vi "init.vi"(8 "error in":errorcluster, 10 "TBM module configuration in":refnum<class "TBM module configuration.lvclass">, 11 "fixed channel runtime in":refnum<class "control module runtime.lvclass">) -> (0 "error out":errorcluster, 1 "data allocations":T1, 2 "execution settings":T4, 3 "fixed channel runtime out":refnum<class "control module runtime.lvclass">)   [LabVIEW 2013, in "control module runtime.lvclass"]
doc: "Provides an interface for initializing a module at runtime. While this interface performs no operations, a child should provide an override which may open any necessary references or sessions, allocate necessary memory, and perform any final configuration validataion before providing the full configuration <b>execution data</b> to the calling process."
uses:
  control module runtime.lvclass
  <vilib>/NI/Tag Bus Module Framework/module configuration/TBM module configuration.lvclass
  <vilib>/NI/Tag Bus Module Framework/runtime/execution settings.ctl
  <vilib>/NI/Tag Bus Module Framework/channel/data tables.ctl
  <vilib>/NI/Tag Bus/dictionary/data dictionary.lvclass
  <vilib>/NI/Tag Bus/dictionary table pair.ctl
  <vilib>/NI/Tag Bus/table/data table.ctl
  configuration/control module configuration.lvclass
  <vilib>/NI/Tag Bus Module Framework/channel/TBM channel.lvclass
  <vilib>/NI/Tag Bus Module Framework/runtime/TBM module execution interface.lvclass
  <vilib>/NI/Tag Bus/tag bus.lvlib
  <vilib>/NI/Tag Bus/table/data table.lvlib
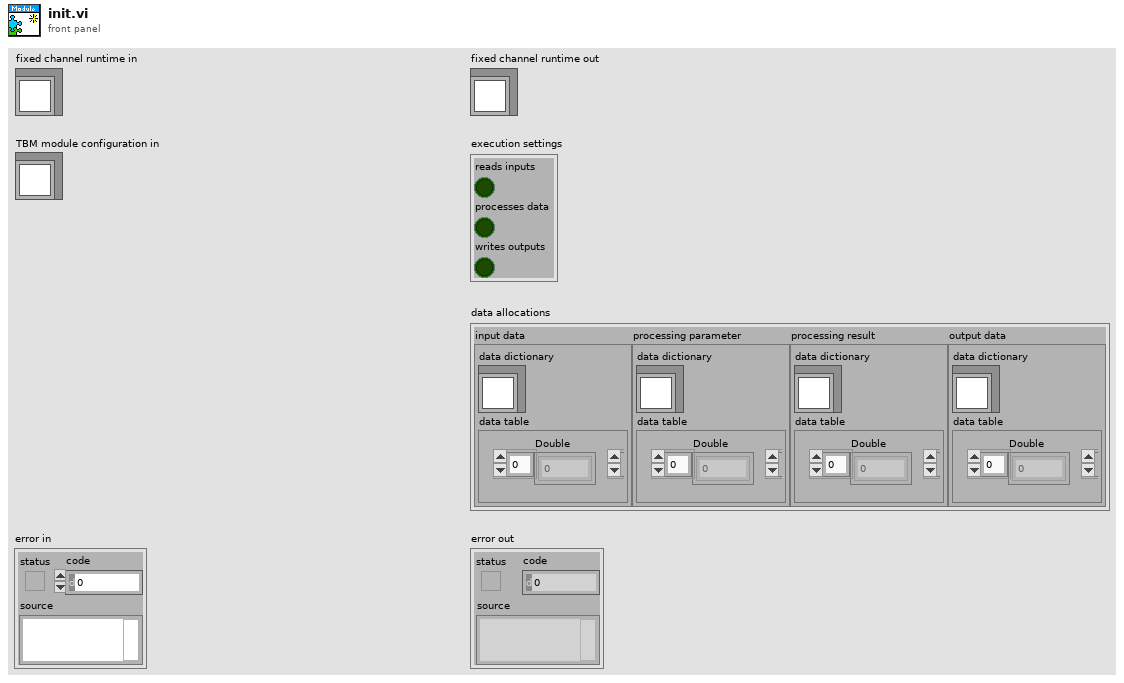
[diagram p1: front panel]
types:
  T1 = typedef "TBM channel.lvclass/data tables.ctl" = cluster{"input data":T2, "processing parameter":T2, "processing result":T2, "output data":T2}
  T2 = typedef "tag bus.lvlib/dictionary table pair.ctl" = cluster{"data dictionary":refnum<class "data dictionary.lvclass">, "data table":T3}
  T3 = typedef "tag bus.lvlib/data table.lvlib/data table.ctl" = cluster{"Double":dbl[], "Single":sgl[], "I64":i64[], "I32":i32[], "I16":i16[], "I8":i8[], "U64":u64[], "U32":u32[], "U16":u16[], "U8":u8[], "Boolean":bool[], "String":string[], "Array of Double":cluster{"DBL Array":dbl[]}[], "Array of Single":cluster{"SGL Array":sgl[]}[], "Array of I64":cluster{"I64 Array":i64[]}[], "Array of I32":cluster{"I32 Array":i32[]}[], "Array of I16":cluster{"I16 Array":i16[]}[], "Array of I8":cluster{"I8 Array":i8[]}[], "Array of U64":cluster{"U64 Array":u64[]}[], "Array of U32":cluster{"U32 Array":u32[]}[], "Array of U16":cluster{"U16 Array":u16[]}[], "Array of U8":cluster{"U8 Array":u8[]}[], "Array of Boolean":cluster{"Boolean Array":bool[]}[], "Array of String":cluster{"String Array":string[]}[]}
  T4 = typedef "TBM module execution interface.lvclass/execution settings.ctl" = cluster{"reads inputs":bool, "processes data":bool, "writes outputs":bool}
  T5 = typedef "control module runtime.lvclass/Channel Run Time Mapping Info.ctl" = cluster{"Channel Indicies":i32[], "Channel Names":string[]}
  T6 = typedef "TBM channel.lvclass/channel classification.ctl" = enum16{"input data", "output data", "processing parameter", "processing result"}
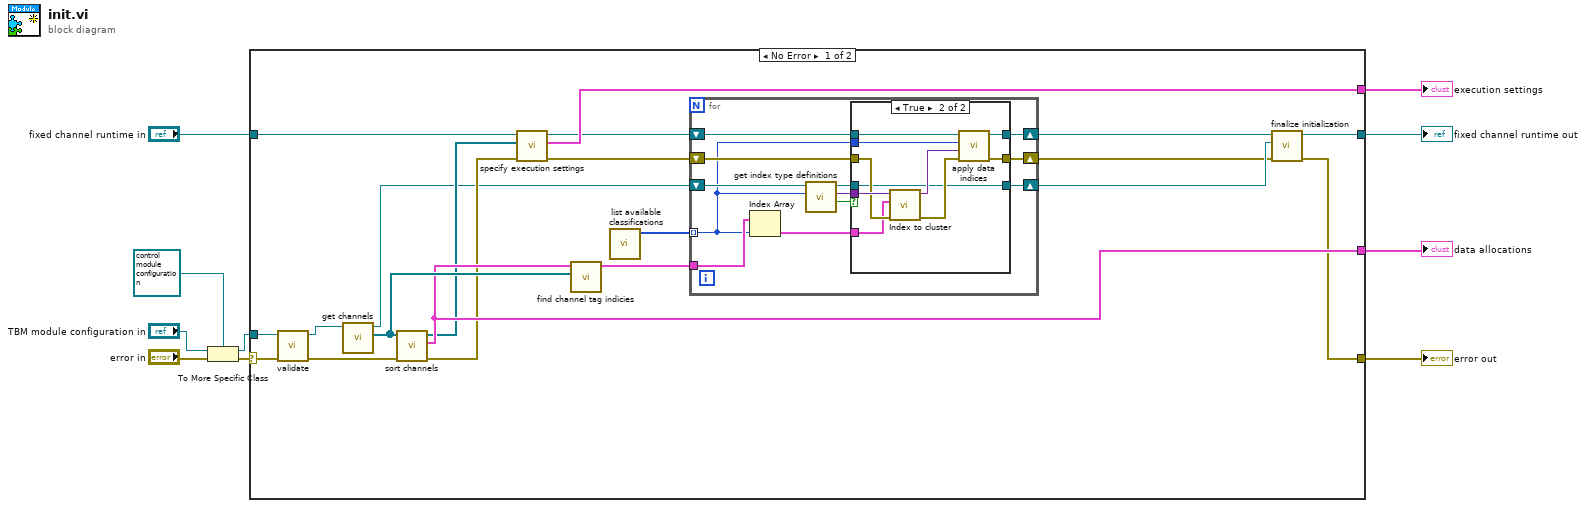
[diagram p0: block diagram]
diagram:
  n1 = To More Specific Class(target class=refnum<class "control module configuration.lvclass"> refnum ("Synchronous module configuration"), reference="TBM module configuration in", error in="error in") -> (specific class reference=w1:refnum<class "control module configuration.lvclass">, error out=w2:errorcluster)
  n2 = case shown="No Error" w2 {
    selector: w2 -> [w29 w56]
    tunnel: w1 -> [w28 _]
    tunnel: "fixed channel runtime in" -> [w22 w57]
    tunnel: [w24 w57] -> w8
    tunnel: [w23 w56] -> w7
    tunnel: [w25 _] -> w5
    tunnel: [w21 _] -> w6
    frame No Error {
      n3 = call-dynamic "validate.vi"("error in"=w29, "fixed channel configuration in"=w28) -> ("error out"=w30:errorcluster, "fixed channel configuration out"=w27:refnum<class "control module configuration.lvclass">)  [unwired: 8 in]
      n4 = call-dynamic "get channels.vi"("fixed channel configuration in"=w27) -> ("channels"=w26:refnum<class "TBM channel.lvclass">[], "fixed channel configuration out"=w16:refnum<class "control module configuration.lvclass">)  [unwired: 9 in]
      n5 = call <vilib>:"sort channels.vi"("error in"=w30, "channels in"=w26) -> ("error out"=w19:errorcluster, "data allocations"=w25:T1, "channels out"=w20:refnum<class "TBM channel.lvclass">[])  [unwired: 7 in]
      n6 = call-dynamic "specify execution settings.vi"("error in"=w19, "channels"=w20, "fixed channel runtime in"=w22) -> ("error out"=w12:errorcluster, "execution settings"=w21:T4, "fixed channel runtime out"=w18:refnum<class "control module runtime.lvclass">)  [unwired: 6 in]
      n7 = call "find channel tag indicies.vi"("channels"=w26, "data allocations"=w25) -> ("classified indices"=w11:T5[])  [unwired: 9 in]
      n8 = call <vilib>:"list available classifications.vi"() -> ("supported types"=w17:T6[])  [unwired: 11 in]
      n9 = for {
        shift-right: [w38] -> w15
        shift-left: w18 -> [w37]
        tunnel: w17 -> [w32] mode=indexing
        shift-right: [w39] -> w14
        shift-left: w16 -> [w42]
        shift-right: [w36] -> w13
        shift-left: w12 -> [w35]
        tunnel: w11 -> [w33]
        n10 = Index Array(array=w33, index=w32) -> (element=w31:T5)
        n11 = call-dynamic "get index type definitions.vi"("channel classification"=w32, "fixed channel configuration in"=w42) -> ("valid?"=w41:bool, "index cluster"=w34:variant, "fixed channel configuration out"=w40:refnum<class "control module configuration.lvclass">)  [unwired: 7 in]
        n12 = case shown="True" w41 {
          tunnel: w40 -> [w45 w47]
          tunnel: [w45 w47] -> w39
          tunnel: [w44 w55] -> w38
          tunnel: w37 -> [w44 w54]
          tunnel: [w43 w53] -> w36
          tunnel: w35 -> [w43 w50]
          tunnel: w32 -> [_ w52]
          tunnel: w34 -> [_ w51]
          tunnel: w31 -> [_ w46]
          frame False {
          }
          frame True {
            n13 = call "Index to cluster.vi"("error in"=w50, "Input Mapping Info"=w46, "Variant in"=w51) -> ("error out"=w49:errorcluster, "Variant out"=w48:variant)  [unwired: 7 in]
            n14 = call-dynamic "apply data indices.vi"("error in"=w49, "index cluster"=w48, "channel classification"=w52, "fixed channel runtime in"=w54) -> ("error out"=w53:errorcluster, "fixed channel runtime out"=w55:refnum<class "control module runtime.lvclass">)  [unwired: 6 in]
          }
        }
      }
      n15 = call-dynamic "finalize initialization.vi"("error in"=w13, "configuration in"=w14, "fixed channel runtime in"=w15) -> ("error out"=w23:errorcluster, "fixed channel runtime out"=w24:refnum<class "control module runtime.lvclass">)  [unwired: 7 in]
    }
    frame Error {
    }
  }
  "error out" <- w7
  "fixed channel runtime out" <- w8
  "execution settings" <- w6
  "data allocations" <- w5
